vi "Transtake Teleop.vi"   [LabVIEW 2019]
uses:
  Implementation/Intake & Transfer Operations.ctl
types:
  T1 = typedef "Intake & Transfer Operations.ctl" = enum16{"Reserve", "Read Current", "Ready"}
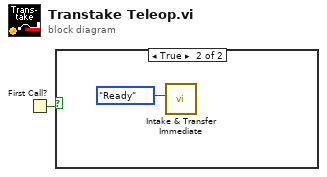
[diagram p0: block diagram]
diagram:
  n1 = First Call?() -> (First Call?: T/F=w1:bool)
  n2 = case shown="True" w1 {
    frame False {
    }
    frame True {
      n3 = call "Intake & Transfer Immediate.vi"("Operation"=Intake_&_Transfer_Operations."Ready") -> ()  [unwired: 10 in, 1 out]
    }
  }
